vi "Pull Info From XNET Database.vi"(8 "error in":errorcluster, 10 "Frame Configuration":T1 {"CRCConfiguration"."FinalXorValue" format="%0x"; "CRCConfiguration"."InitialCRC" format="%0x"; "CRCConfiguration"."Polynomial" format="%0x"; "CRC"."Data Type" items=["Signed", "Unsigned", "IEEE Float"]; "Rolling Counter"."Data Type" items=["Signed", "Unsigned", "IEEE Float"]; "Input Channels"."Data Type" items=["Signed", "Unsigned", "IEEE Float"]}, 11 "Parent Ref":T5=18446744073709551615 format="%.0x") -> (0 "error out":errorcluster, 2 "Frame Configuration":T1 {"CRCConfiguration"."FinalXorValue" format="%0x"; "CRCConfiguration"."InitialCRC" format="%0x"; "CRCConfiguration"."Polynomial" format="%0x"; "CRC"."Data Type" items=["Signed", "Unsigned", "IEEE Float"]; "Rolling Counter"."Data Type" items=["Signed", "Unsigned", "IEEE Float"]; "Input Channels"."Data Type" items=["Signed", "Unsigned", "IEEE Float"]}, 3 "Item Ref out":T5 format="%.0x")   [LabVIEW 2021, in "LIN Frame Protection Addon System Explorer.lvlib"]
uses:
  LIN Frame Protection Addon System Explorer.lvlib
  Shared/Types/FrameConfiguration.ctl
  Shared/Types/InputChannelConfiguration.ctl
  Shared/Types/Protection Type.ctl
  Shared/Types/CRCConfiguration.ctl
  <vilib>/NI VeriStand/Custom Device API/Custom Device Item Ref.ctl
  NationalInstruments.VeriStand.SystemStorage
  NationalInstruments.VeriStand
  <vilib>/NI VeriStand/Custom Device API/Custom Device API.lvlib
  <vilib>/NI VeriStand/Custom Device Tools/Custom Device Utility Library/Custom Device Utility Library.lvlib
  <resource>/objmgr/xnet.rc
  Shared/LIN Frame Protection Addon Shared.lvlib
panel:
  out "Value":string
  out "Array":string[](array[string])
  out "CycleTime":dbl[](array[numeric])
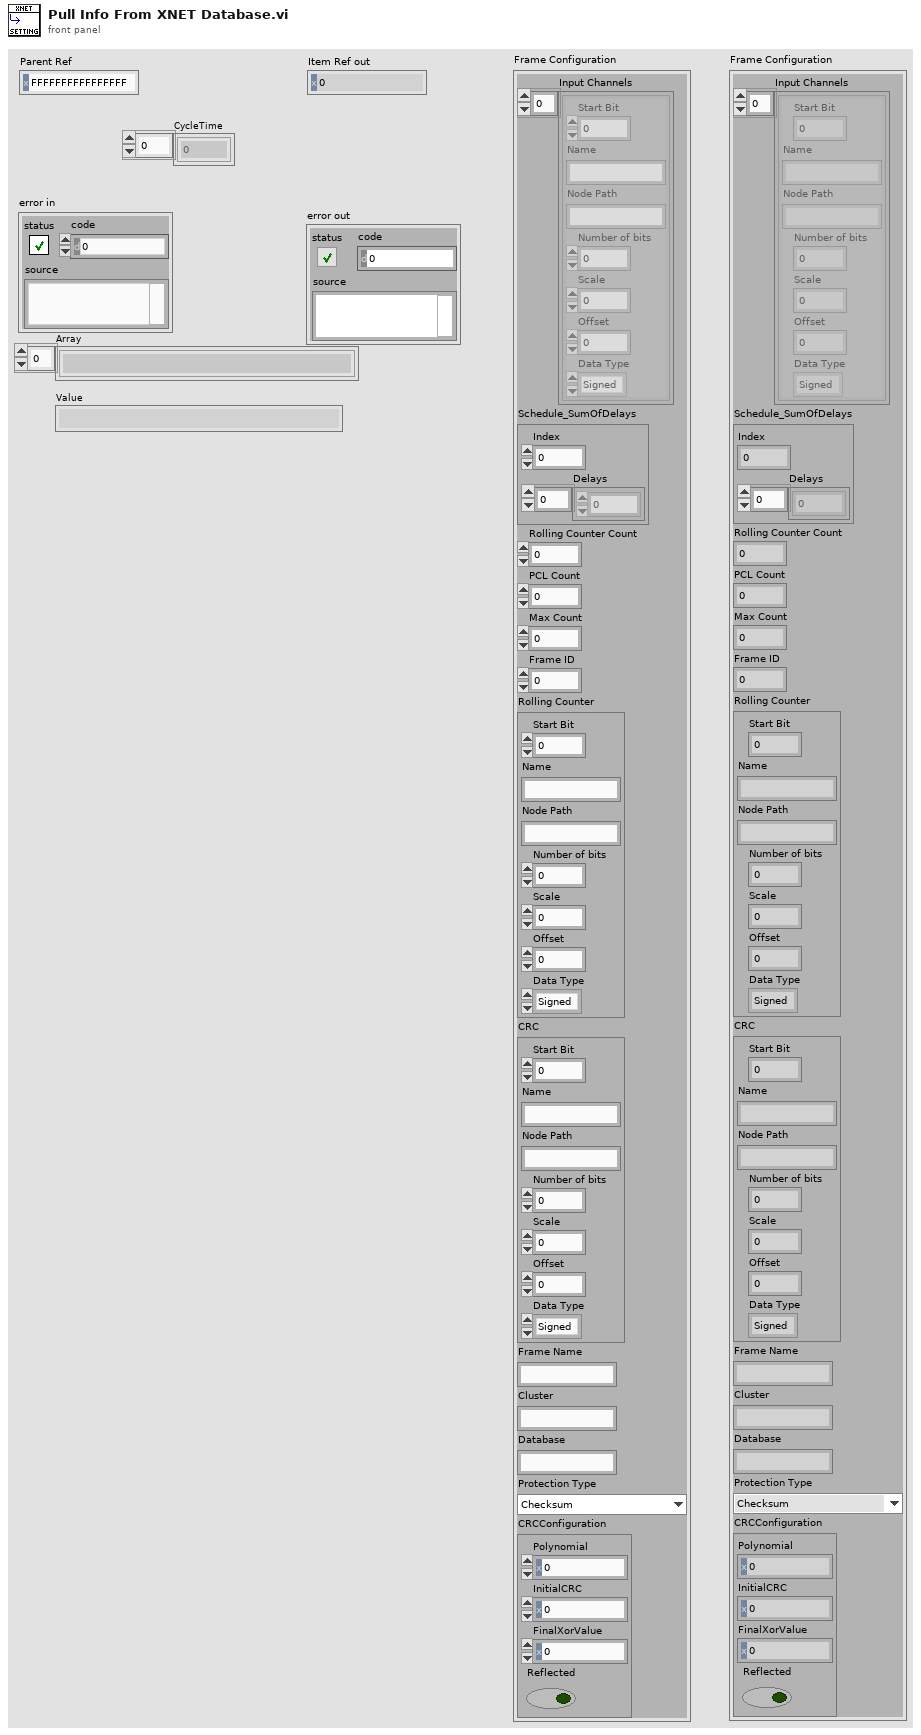
[diagram p1: front panel]
types:
  T1 = typedef "LIN Frame Protection Addon Shared.lvlib/FrameConfiguration.ctl" = cluster{"Input Channels":T2[], "Schedule_SumOfDelays":cluster{"Index":i32, "Delays":dbl[]}, "Rolling Counter Count":dbl, "PCL Count":u64, "Max Count":dbl, "Frame ID":u32, "Rolling Counter":T2, "CRC":T2, "Frame Name":string, "Cluster":string, "Database":string, "Protection Type":T3, "CRCConfiguration":T4}
  T2 = typedef "LIN Frame Protection Addon Shared.lvlib/InputChannelConfiguration.ctl" = cluster{"Start Bit":i32, "Name":string, "Node Path":string, "Number of bits":i32, "Scale":dbl, "Offset":dbl, "Data Type":u32}
  T3 = typedef "LIN Frame Protection Addon Shared.lvlib/Protection Type.ctl" = enum16{"Checksum", "CRC-8", "CRC-16", "CRC-32", "None (Counter Only)"}
  T4 = typedef "LIN Frame Protection Addon Shared.lvlib/CRCConfiguration.ctl" = cluster{"Polynomial":u64, "InitialCRC":u64, "FinalXorValue":u64, "Reflected":bool}
  T5 = typedef "Custom Device API.lvlib/Custom Device Item Ref.ctl" = u64
  T6 = typedef "Custom Device API.lvlib/Custom Device Pointer.ctl" = refnum<k24>
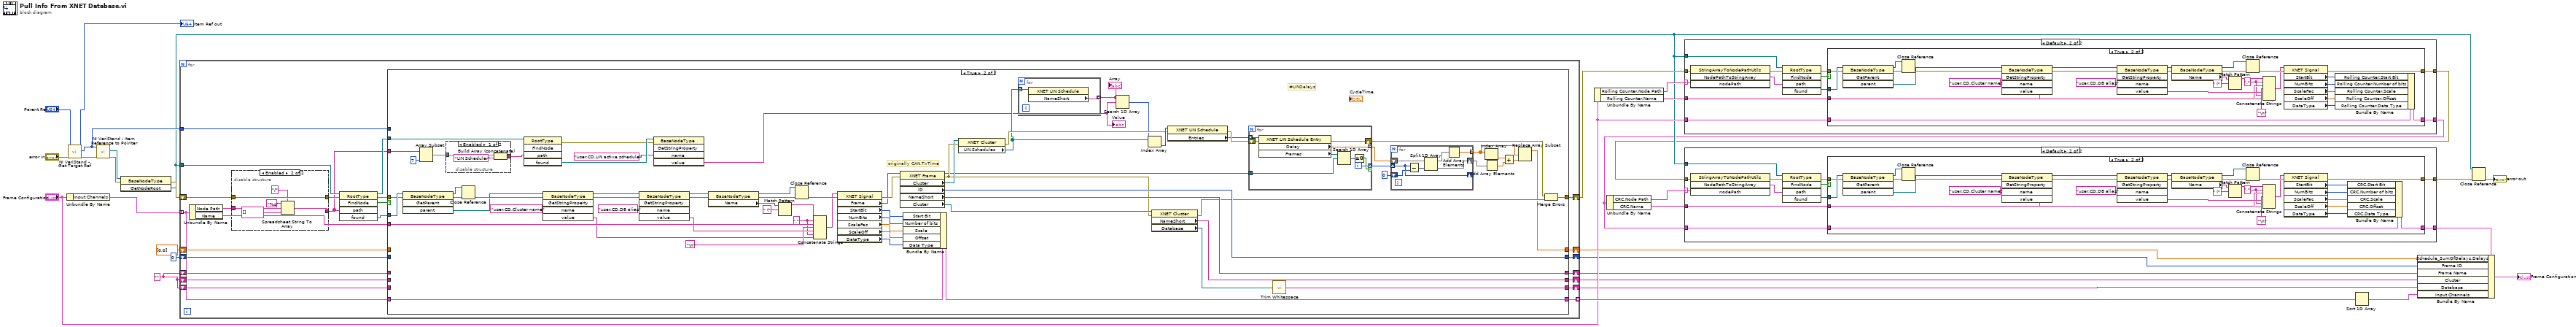
[diagram p0: block diagram]
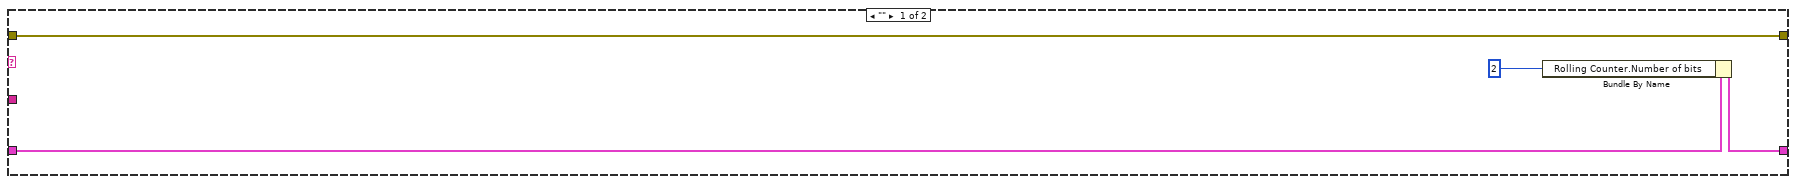
[diagram p2: hidden frame]
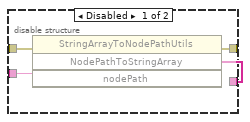
[diagram p4: hidden frame]
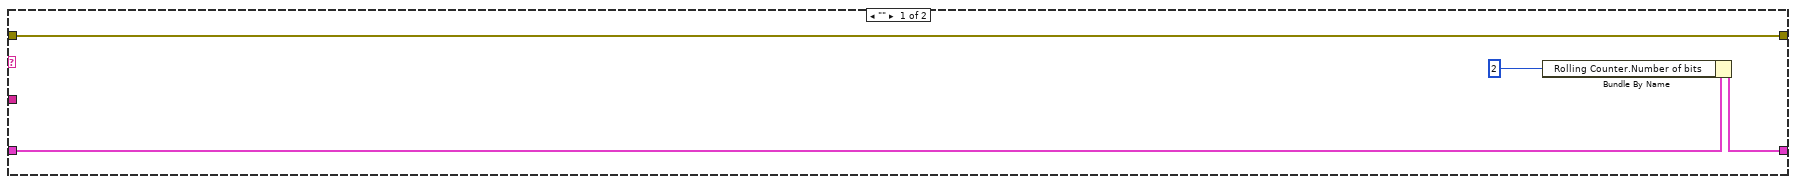
[diagram p7: hidden frame]
diagram:
  w14 = "" ("NameShort")
  n1 = Unbundle By Name("Frame Configuration") -> ("Input Channels"=w29:T2[])
  n2 = call <vilib>:"NI VeriStand - Get Target Ref.vi"("error in"="error in", "Item Ref in"="Parent Ref") -> ("error out"=w30:errorcluster, "Target Ref"=w10:T5, "Item Ref out"=→"Item Ref out":T5)  [unwired: 6 in, 1 out]
  n3 = call <vilib>:"NI VeriStand - Item Reference to Pointer.vi"("error in (no error)"=w30, "Item Ref in"=w10) -> ("error out"=w25:errorcluster, "Node Pointer"=w26:T6)  [unwired: 6 in, 2 out]
  n4 = invoke class="BaseNodeType" method="GetNodeRoot"(reference=w26, error in=w25) -> (error out=w24:errorcluster, "GetNodeRoot"=w5:refnum<k24>)  [unwired: 1 in, 1 out]
  n5 = for {
    tunnel: w5 -> [w50]
    shift-right: [w52] -> w18
    shift-left: w24 -> [w56]
    tunnel: w29 -> [w47] mode=indexing
    tunnel: [w46] -> w23 mode=indexing
    shift-right: [w45] -> w19
    shift-left: dbl[] [0.0] ("CAN.TxTime") -> [w44]
    shift-right: [w43] -> w15
    shift-left: u32 0 ("ID") -> [w42]
    shift-right: [w41] -> w11
    shift-left: w14 -> [w40]
    shift-right: [w39] -> w12
    shift-left: w14 -> [w37]
    shift-right: [w38] -> w13
    shift-left: w14 -> [w36]
    tunnel: w10 -> [w35]
    n6 = Unbundle By Name(w47) -> ("Node Path"=w51:string, "Name"=w48:string)
    n7 = disable-structure shown="Enabled" {
      disable-tunnel: w56 -> [w60 w66]
      disable-tunnel: [w59 w66] -> w55
      disable-tunnel: w51 -> [w58 w62]
      disable-tunnel: [w57 w64] -> w33
      frame Disabled {
        n8 = invoke class="StringArrayToNodePathUtils" method="NodePathToStringArray"(error in=w60, "nodePath"=w58) -> (error out=w59:errorcluster, "NodePathToStringArray"=w57:string[])  [unwired: 2 in, 2 out]
      }
      frame Enabled {
        n9 = Spreadsheet String To Array(delimiter (Tab)="/", format string="%s", spreadsheet string=w62, array type (2D Dbl)=string[] [] ("Node Path")) -> (array=w64:string[])
      }
    }
    n10 = invoke class="RootType" method="FindNode"(reference=w50, error in=w55, "path"=w33) -> (reference out=w34:refnum<k24>, error out=w49:errorcluster, "FindNode"=w53:bool, "found"=w54:refnum<k24>)  [unwired: 2 in, 1 out]
    n11 = case shown="True" w53 {
      tunnel: w49 -> [w73 w142]
      tunnel: w54 -> [_ w143]
      tunnel: [w73 w98] -> w52
      tunnel: w48 -> [_ w140]
      tunnel: w47 -> [w72 w139]
      tunnel: [w72 w135] -> w46
      tunnel: [w71 w88] -> w45
      tunnel: w44 -> [w71 _]
      tunnel: [w70 w123] -> w43
      tunnel: w42 -> [w70 _]
      tunnel: [w69 w122] -> w41
      tunnel: w40 -> [w69 _]
      tunnel: [w68 w120] -> w39
      tunnel: [w67 w118] -> w38
      tunnel: w37 -> [w68 _]
      tunnel: w36 -> [w67 _]
      tunnel: w35 -> [_ _]
      tunnel: w34 -> [_ w82]
      tunnel: w33 -> [_ w81]
      frame False {
      }
      frame True {
        w107 = "." ("string")
        # "#LINDelays"
        # "originally CAN.TxTime"
        n12 = invoke class="BaseNodeType" method="GetParent"(reference=w143, error in=w142) -> (reference out=w130:refnum<k24>, error out=w131:errorcluster, "parent"=w110:refnum<k24>)  [unwired: 2 in, 1 out]
        n13 = Array Subset(array=w81, length=7) -> (w80:string[])  [unwired: 1 in]
        n14 = disable-structure shown="Enabled" {
          disable-tunnel: w80 -> [w146 w147]
          disable-tunnel: [w145 w147] -> w78
          frame Enabled {
            n15 = Build Array (concatenate)(w146, "LIN Scheduler" ("array")) -> (w145:string[])
          }
          frame Disabled {
          }
        }
        n16 = Close Reference(reference=w130, error in (no error)=w131) -> (error out=w112:errorcluster)
        n17 = invoke class="RootType" method="FindNode"(reference=w82, "path"=w78) -> (error out=w76:errorcluster, "found"=w77:refnum<k24>)  [unwired: 3 in, 3 out]
        n18 = invoke class="BaseNodeType" method="GetStringProperty"(reference=w110, error in=w112, "name"="user.CD.Cluster name") -> (reference out=w109:refnum<k24>, error out=w111:errorcluster, "value"=w106:string)  [unwired: 2 in, 2 out]
        n19 = invoke class="BaseNodeType" method="GetStringProperty"(reference=w109, error in=w111, "name"="user.CD.DB alias") -> (reference out=w114:refnum<k24>, error out=w128:errorcluster, "value"=w108:string)  [unwired: 2 in, 2 out]
        n20 = invoke class="BaseNodeType" method="GetStringProperty"(reference=w77, error in=w76, "name"="user.CD.LIN active schedule" ("Property Name")) -> ("value"=w74:string)  [unwired: 2 in, 4 out]
        "Value" <- w74
        n21 = property class="BaseNodeType"(reference=w114, error in=w128) -> (reference out=w129:refnum<k24>, error out=w127:errorcluster, "Name"=w126:string)
        n22 = Match Pattern(string=w126, regular expression=" (") -> (before substring=w117:string)  [unwired: 1 in, 3 out]
        n23 = Close Reference(reference=w129, error in (no error)=w127) -> (error out=w132:errorcluster)
        n24 = Concatenate Strings(w117, w107, w140, "\n", w108, w107, w106) -> (w105:string)
        n25 = property class="XNET Signal"(reference=w105, error in=w132) -> (error out=w133:errorcluster, "Frame"=w115:refnum<k21>, "StartBit"=w134:u32, "NumBits"=w138:u32, "ScaleFac"=w136:dbl, "ScaleOff"=w137:dbl, "DataType"=w124:u32)  [unwired: 1 out]
        n26 = property class="XNET Frame"(reference=w115, error in=w133) -> (reference out=w92:refnum<k21>, error out=w100:errorcluster, "Cluster"=w104:refnum<k21>, "ID"=w123:u32, "NameShort"=w122:string, "Cluster"=w121:refnum<k21>)
        n27 = Bundle By Name(cluster=w139, "Start Bit"=w134, "Number of bits"=w138, "Scale"=w136, "Offset"=w137, "Data Type"=w124) -> (w135:T2)
        n28 = property class="XNET Cluster"(reference=w104, error in=w100) -> (error out=w99:errorcluster, "LIN.Schedules"=w95:refnum<k21>[])  [unwired: 1 out]
        n29 = for {
          tunnel: [w156] -> w94 mode=indexing
          tunnel: w95 -> [w155] mode=indexing
          n30 = property class="XNET LIN Schedule"(reference=w155) -> ("NameShort"=w156:string)  [unwired: 1 in, 2 out]
        }
        "Array" <- w94
        n31 = Search 1D Array(1D array=w94, element=w74) -> (index of element=w93:i32)  [unwired: 1 in]
        n32 = Index Array(array=w95, index=w93) -> (element=w103:refnum<k21>)
        n33 = property class="XNET Cluster"(reference=w121, error in=w100) -> (error out=w97:errorcluster, "NameShort"=w120:string, "Database"=w119:refnum<k21>)  [unwired: 1 out]
        n34 = property class="XNET LIN Schedule"(reference=w103, error in=w99) -> (error out=w102:errorcluster, "Entries"=w101:refnum<k21>[])  [unwired: 1 out]
        n35 = for {
          tunnel: w101 -> [w162] mode=indexing
          tunnel: [w164] -> w87 mode=indexing
          shift-right: [w163] -> w96
          shift-left: w102 -> [w165]
          tunnel: w92 -> [w160]
          tunnel: [w158] -> w86 mode=indexing if=w157
          i -> [w158]
          n36 = property class="XNET LIN Schedule Entry"(reference=w162, error in=w165) -> (error out=w163:errorcluster, "Delay"=w164:dbl, "Frames"=w161:refnum<k21>[])  [unwired: 1 out]
          n37 = Search 1D Array(1D array=w161, element=w160) -> (index of element=w159:i32)  [unwired: 1 in]
          n38 = Greater Or Equal To 0?(x=w159) -> (x >= 0?=w157:bool)
        }
        n39 = call <vilib>:"Trim Whitespace.vi"("string"=w119) -> ("trimmed string"=w118:string)  [unwired: 1 in]
        n40 = for {
          tunnel: w86 -> [w148] mode=indexing
          shift-right: [w153] -> w84
          shift-left: w87 -> [w154]
          tunnel: [w151] -> w85 mode=indexing
          shift-right: [w148] -> _
          shift-left: 0 -> [w150]
          n41 = Subtract(x=w148, y=w150) -> (x-y=w149:i32)
          n42 = Split 1D Array(array=w154, index=w149) -> (first subarray=w152:dbl[], second subarray=w153:dbl[])
          n43 = Add Array Elements(numeric array=w152) -> (sum=w151:dbl)
        }
        n44 = Index Array(array=w85) -> (element=w91:dbl)  [unwired: 1 in]
        n45 = Add Array Elements(numeric array=w84) -> (sum=w89:dbl)
        n46 = Add(x=w91, y=w89) -> (x+y=w90:dbl)
        n47 = Replace Array Subset(array=w85, new element=w90) -> (w88:dbl[])  [unwired: 1 in]
        n48 = Merge Errors(w96, w97) -> (w98:errorcluster)
      }
    }
  }
  n49 = Unbundle By Name("Frame Configuration") -> ("Rolling Counter.Node Path"=w8:string, "Rolling Counter.Name"=w9:string)
  n50 = case shown="Default" w8 {
    selector: w8 -> [_ w170]
    tunnel: w9 -> [_ w176]
    tunnel: w5 -> [_ w175]
    tunnel: w18 -> [w169 w174]
    tunnel: [w169 w173] -> w4
    tunnel: "Frame Configuration" -> [w168 w172]
    tunnel: [w167 w171] -> w2
    frame "" {
      n51 = Bundle By Name(cluster=w168, "Rolling Counter.Number of bits"=u32 2 ("Rolling Counter Length")) -> (w167:T1)
    }
    frame Default {
      n52 = invoke class="StringArrayToNodePathUtils" method="NodePathToStringArray"(error in=w174, "nodePath"=w170) -> (error out=w181:errorcluster, "NodePathToStringArray"=w178:string[])  [unwired: 2 in, 2 out]
      n53 = invoke class="RootType" method="FindNode"(reference=w175, error in=w181, "path"=w178) -> (error out=w177:errorcluster, "FindNode"=w179:bool, "found"=w180:refnum<k24>)  [unwired: 2 in, 2 out]
      n54 = case shown="True" w179 {
        tunnel: w177 -> [w183 w214]
        tunnel: w180 -> [_ w215]
        tunnel: [w183 w203] -> w173
        tunnel: w176 -> [_ w210]
        tunnel: w172 -> [w182 w209]
        tunnel: [w182 w207] -> w171
        frame False {
        }
        frame True {
          w186 = "." ("string")
          n55 = invoke class="BaseNodeType" method="GetParent"(reference=w215, error in=w214) -> (reference out=w204:refnum<k24>, error out=w205:errorcluster, "parent"=w188:refnum<k24>)  [unwired: 2 in, 1 out]
          n56 = Close Reference(reference=w204, error in (no error)=w205) -> (error out=w190:errorcluster)
          n57 = invoke class="BaseNodeType" method="GetStringProperty"(reference=w188, error in=w190, "name"="user.CD.Cluster name") -> (reference out=w187:refnum<k24>, error out=w189:errorcluster, "value"=w185:string)  [unwired: 2 in, 2 out]
          n58 = invoke class="BaseNodeType" method="GetStringProperty"(reference=w187, error in=w189, "name"="user.CD.DB alias") -> (reference out=w200:refnum<k24>, error out=w202:errorcluster, "value"=w211:string)  [unwired: 2 in, 2 out]
          n59 = property class="BaseNodeType"(reference=w200, error in=w202) -> (reference out=w199:refnum<k24>, error out=w201:errorcluster, "Name"=w197:string)
          n60 = Match Pattern(string=w197, regular expression=" (") -> (before substring=w196:string)  [unwired: 1 in, 3 out]
          n61 = Close Reference(reference=w199, error in (no error)=w201) -> (error out=w206:errorcluster)
          n62 = Concatenate Strings(w196, w186, w210, "\n", w211, w186, w185) -> (w184:string)
          n63 = property class="XNET Signal"(reference=w184, error in=w206) -> (error out=w203:errorcluster, "StartBit"=w208:u32, "NumBits"=w195:u32, "ScaleFac"=w194:dbl, "ScaleOff"=w193:dbl, "DataType"=w192:u32)  [unwired: 1 out]
          n64 = Bundle By Name(cluster=w209, "Rolling Counter.Start Bit"=w208, "Rolling Counter.Number of bits"=w195, "Rolling Counter.Scale"=w194, "Rolling Counter.Offset"=w193, "Rolling Counter.Data Type"=w192) -> (w207:T1)
        }
      }
    }
  }
  n65 = Unbundle By Name(w2) -> ("CRC.Node Path"=w7:string, "CRC.Name"=w6:string)
  n66 = case shown="Default" w7 {
    selector: w7 -> [_ w220]
    tunnel: w6 -> [_ w226]
    tunnel: w5 -> [_ w225]
    tunnel: w4 -> [w219 w224]
    tunnel: [w219 w223] -> w3
    tunnel: w2 -> [w218 w222]
    tunnel: [w217 w221] -> w1
    frame "" {
      n67 = Bundle By Name(cluster=w218, "Rolling Counter.Number of bits"=u32 2 ("Rolling Counter Length")) -> (w217:T1)
    }
    frame Default {
      n68 = invoke class="StringArrayToNodePathUtils" method="NodePathToStringArray"(error in=w224, "nodePath"=w220) -> (error out=w231:errorcluster, "NodePathToStringArray"=w228:string[])  [unwired: 2 in, 2 out]
      n69 = invoke class="RootType" method="FindNode"(reference=w225, error in=w231, "path"=w228) -> (error out=w227:errorcluster, "FindNode"=w229:bool, "found"=w230:refnum<k24>)  [unwired: 2 in, 2 out]
      n70 = case shown="True" w229 {
        tunnel: w227 -> [w233 w264]
        tunnel: w230 -> [_ w265]
        tunnel: [w233 w253] -> w223
        tunnel: w226 -> [_ w260]
        tunnel: w222 -> [w232 w259]
        tunnel: [w232 w257] -> w221
        frame False {
        }
        frame True {
          w236 = "." ("string")
          n71 = invoke class="BaseNodeType" method="GetParent"(reference=w265, error in=w264) -> (reference out=w254:refnum<k24>, error out=w255:errorcluster, "parent"=w238:refnum<k24>)  [unwired: 2 in, 1 out]
          n72 = Close Reference(reference=w254, error in (no error)=w255) -> (error out=w240:errorcluster)
          n73 = invoke class="BaseNodeType" method="GetStringProperty"(reference=w238, error in=w240, "name"="user.CD.Cluster name") -> (reference out=w237:refnum<k24>, error out=w239:errorcluster, "value"=w235:string)  [unwired: 2 in, 2 out]
          n74 = invoke class="BaseNodeType" method="GetStringProperty"(reference=w237, error in=w239, "name"="user.CD.DB alias") -> (reference out=w250:refnum<k24>, error out=w252:errorcluster, "value"=w261:string)  [unwired: 2 in, 2 out]
          n75 = property class="BaseNodeType"(reference=w250, error in=w252) -> (reference out=w249:refnum<k24>, error out=w251:errorcluster, "Name"=w247:string)
          n76 = Match Pattern(string=w247, regular expression=" (") -> (before substring=w246:string)  [unwired: 1 in, 3 out]
          n77 = Close Reference(reference=w249, error in (no error)=w251) -> (error out=w256:errorcluster)
          n78 = Concatenate Strings(w246, w236, w260, "\n", w261, w236, w235) -> (w234:string)
          n79 = property class="XNET Signal"(reference=w234, error in=w256) -> (error out=w253:errorcluster, "StartBit"=w258:u32, "NumBits"=w245:u32, "ScaleFac"=w244:dbl, "ScaleOff"=w243:dbl, "DataType"=w242:u32)  [unwired: 1 out]
          n80 = Bundle By Name(cluster=w259, "CRC.Start Bit"=w258, "CRC.Number of bits"=w245, "CRC.Scale"=w244, "CRC.Offset"=w243, "CRC.Data Type"=w242) -> (w257:T1)
        }
      }
    }
  }
  n81 = Sort 1D Array(array=w23) -> (sorted array=w21:T2[])
  n82 = Bundle By Name(cluster=w1, "Schedule_SumOfDelays.Delays"=w19, "Frame ID"=w15, "Frame Name"=w11, "Cluster"=w12, "Database"=w13, "Input Channels"=w21) -> (→"Frame Configuration":T1)
  n83 = Close Reference(reference=w5, error in (no error)=w3) -> (error out=→"error out":errorcluster)
